vi "UnpackFieldsFromBuffer.vi"(8 "error in":errorcluster, 11 "Buffer":u8[](array[numeric])) -> (0 "error out":errorcluster, 3 "Fields Ref Out":T1)   [LabVIEW 2019, in "grpc-lvsupport.lvlib"]
uses:
  grpc-lvsupport.lvlib
  grpcId.ctl
  <vilib>/Utility/error.llb/Error Cluster From Error Code.vi
  <resource>/libgrpc_labview.dll
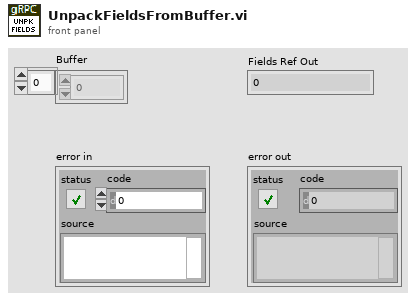
[diagram p1: front panel]
types:
  T1 = typedef "grpc-lvsupport.lvlib/grpcId.ctl" = u64
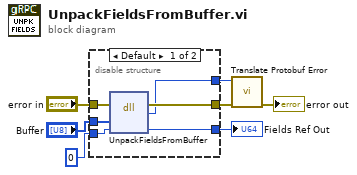
[diagram p0: block diagram]
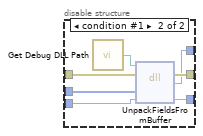
[diagram p2: hidden frame]
diagram:
  n1 = disable-structure shown="Default" {
    disable-tunnel: "error in" -> [w13 w20]
    disable-tunnel: [w12 w19] -> w6
    disable-tunnel: [w11 w17] -> w5
    disable-tunnel: "Buffer" -> [w10 w16]
    disable-tunnel: [w9 w15] -> w2
    disable-tunnel: u64 0 ("elementRef") -> [w8 w14]
    frame condition #0 (active) {
      n2 = dll-call lib="C:/Program Files (x86)/National Instruments/LabVIEW 2024/resource/libgrpc_labview.*" fn="UnpackFieldsFromBuffer"(error in=w13, "buffer"=w10, "elementRef"=w8) -> (error out=w12:errorcluster, "return type"=w9:i32, "elementRef"=w11:u64)  [unwired: 3 in, 1 out]
    }
    frame condition #1 {
      n3 = call "Get Debug DLL Path.vi"() -> ("DLL Path"=w18:path)
      n4 = dll-call lib="?" fn="UnpackFieldsFromBuffer"(path in=w18, error in=w20, "buffer"=w16, "elementRef"=w14) -> (error out=w19:errorcluster, "return type"=w15:i32, "elementRef"=w17:u64)  [unwired: 2 in, 1 out]
    }
  }
  "Fields Ref Out" <- w5
  n5 = call "Translate Protobuf Error.vi"("error in"=w6, "Error Code"=w2) -> ("error out"=→"error out":errorcluster)  [unwired: 9 in]
